vi "Test_Add.vi"(8 "error in (no error)":errorcluster) -> (0 "error out":errorcluster)   [LabVIEW 2021]
uses:
  <vilib>/addons/_JKI Toolkits/Caraya/classes/Assert/Assert Equal Value_Variant.vi
  <vilib>/addons/_JKI Toolkits/Caraya/classes/Test/Test.lvclass
  <vilib>/addons/_JKI Toolkits/Caraya/classes/Assert/Assert.lvclass
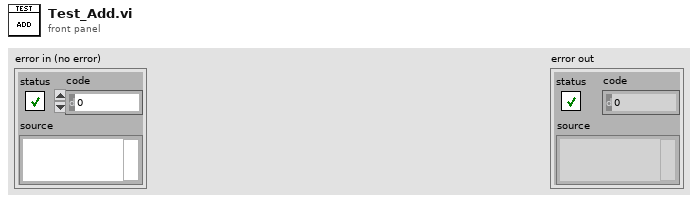
[diagram p1: front panel]
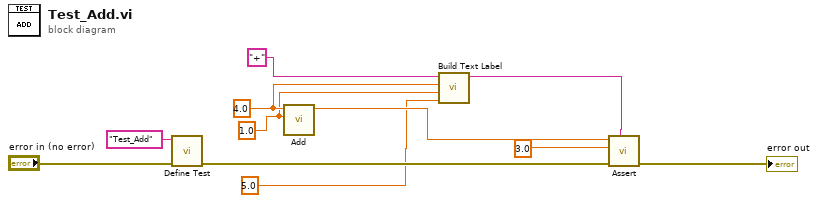
[diagram p0: block diagram]
diagram:
  w3 = 1.0 ("y")
  w5 = 4.0 ("x")
  n1 = call <vilib>:"Define Test.vi"("error in (no error)"="error in (no error)", "Label (VI Title)"="Test_Add") -> ("error out"=w10:errorcluster)  [unwired: 8 in, 1 out]
  n2 = call "Add.vi"("y"=w3, "x"=w5) -> ("x+y"=w11:dbl)  [unwired: 9 in]
  n3 = call "Build Text Label.vi"("x+y"=5.0, "y"=w3, "x"=w5, "Operator"="+" ("chaîne")) -> ("Text Label"=w6:string)  [unwired: 7 in]
  n4 = call-poly <vilib>:"Assert.vi"("Label"=w6, "error in (no error)"=w10, "Y"=3.0 ("x+y"), "X"=w11) -> ("error out"=→"error out":errorcluster)  [unwired: 6 in, 1 out]
